vi "Read_Spill_Intensity.vi"(8 "error in (no error)":errorcluster, 10 "Spill ID":dbl, 11 "Beam in":refnum<class "Beam.lvclass">) -> (0 "error out":errorcluster, 3 "Beam out":refnum<class "Beam.lvclass">)   [LabVIEW 2019, in "Beam.lvclass"]
uses:
  Beam.lvclass
  Beam.lvclass/Beam.ctl
panel:
  in  "Beam Intensity":dbl
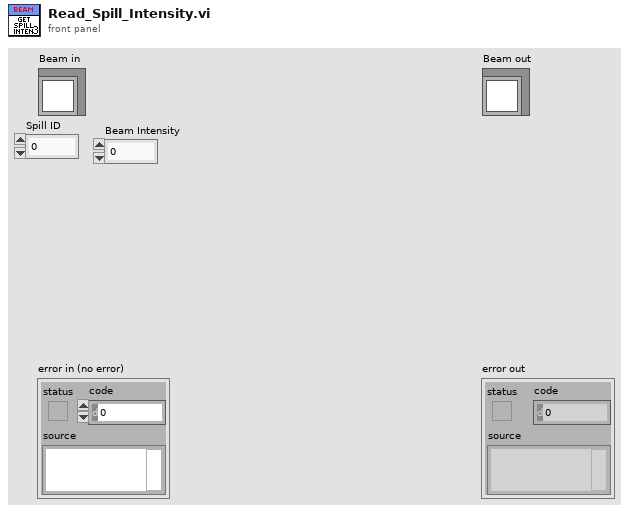
[diagram p1: front panel]
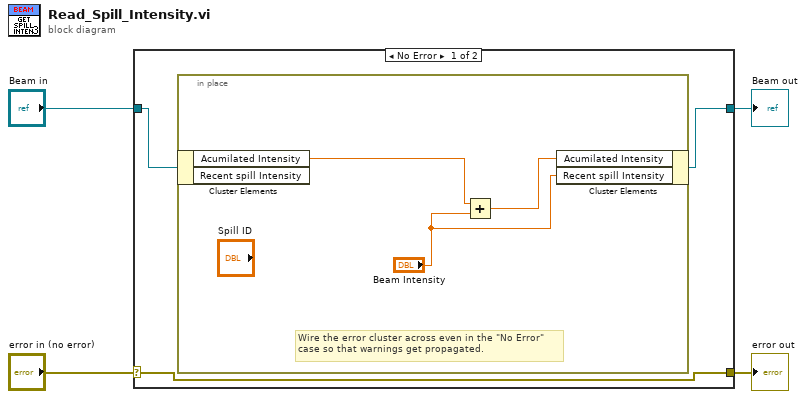
[diagram p0: block diagram]
diagram:
  n1 = case shown="No Error" "error in (no error)" {
    selector: "error in (no error)" -> [w5 w12]
    tunnel: [w5 w12] -> w3
    tunnel: [w6 w11] -> w1
    tunnel: "Beam in" -> [w7 w11]
    frame No Error {
      n2 = in-place {
        # "Wire the error cluster across even in the \"No Error\"\ncase so that warnings get propagated."
        n3 = in-place-cluster #1(w7) -> ("Acumilated Intensity"=w10:dbl)  [unwired: 1 out]
        n4 = Add(x=w10, y="Beam Intensity") -> (x+y=w9:dbl)
        n5 = in-place-cluster #1("Acumilated Intensity"=w9, "Recent spill Intensity"="Beam Intensity") -> (w6:refnum<class "Beam.lvclass">)
      }
    }
    frame Error {
    }
  }
  "error out" <- w3
  "Beam out" <- w1
